vi "NS_GetProperty.vi"(0 "object in":refnum<class "NativeSubTemplate_4x4x4.lvclass">, 5 "error in (no error)":errorcluster) -> (14 "object out":refnum<class "NativeSubTemplate_4x4x4.lvclass">, 15 "property":bool, 19 "error out":errorcluster)   [LabVIEW 2012, in "NativeSubTemplate_4x4x4.lvclass"]
uses:
  NativeSubTemplate_4x4x4.lvclass
  NativeSubTemplate_4x4x4.lvclass/NativeSubTemplate_4x4x4.ctl
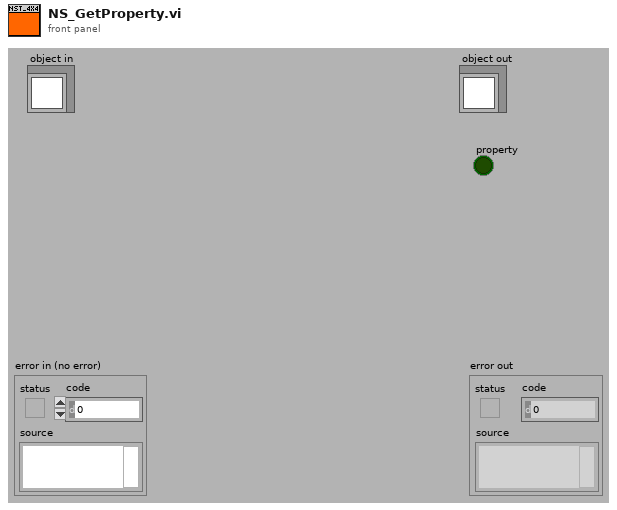
[diagram p1: front panel]
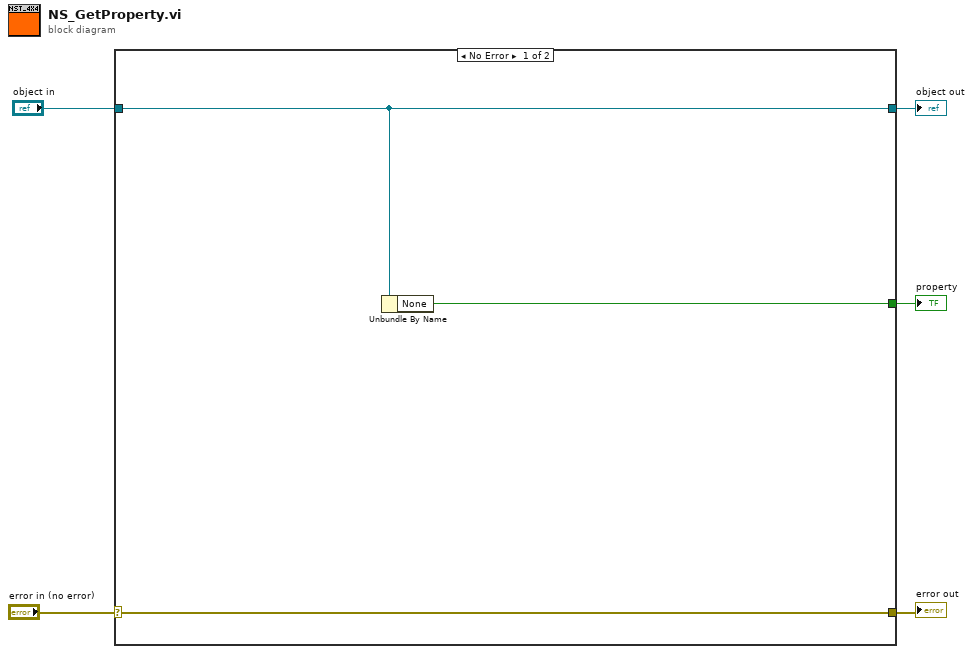
[diagram p0: block diagram]
diagram:
  n1 = case shown="No Error" "error in (no error)" {
    selector: "error in (no error)" -> [w7 w10]
    tunnel: [w7 w10] -> w4
    tunnel: [w6 w9] -> w2
    tunnel: "object in" -> [w6 w9]
    tunnel: [w8 _] -> w1
    frame No Error {
      n2 = Unbundle By Name(w6) -> ("None"=w8:bool)
    }
    frame Error {
    }
  }
  "error out" <- w4
  "object out" <- w2
  "property" <- w1
